vi "Remove Virtual Drive.vi"(8 "error in (no error)":errorcluster, 11 "BuildWorker Controller in":refnum<class "BuildWorker Controller.lvclass">) -> (0 "error out":errorcluster, 3 "BuildWorker Controller out":refnum<class "BuildWorker Controller.lvclass">)   [LabVIEW 2017, in "BuildWorker Controller.lvlib" / "BuildWorker Controller.lvclass"]
uses:
  BuildWorker Controller.lvclass
  BuildWorker Controller.lvclass/BuildWorker Controller.ctl
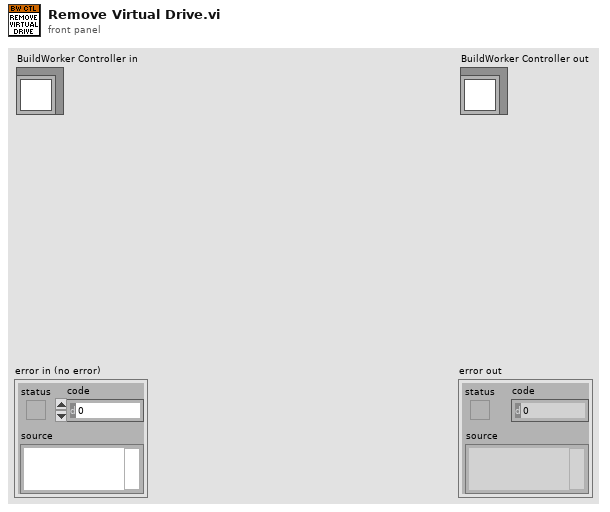
[diagram p1: front panel]
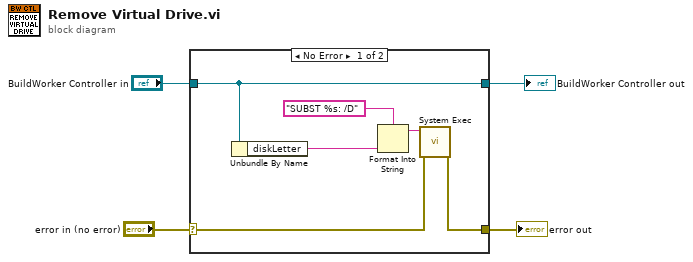
[diagram p0: block diagram]
diagram:
  n1 = case shown="No Error" "error in (no error)" {
    selector: "error in (no error)" -> [w6 w12]
    tunnel: [w5 w12] -> w1
    tunnel: [w10 w11] -> w3
    tunnel: "BuildWorker Controller in" -> [w10 w11]
    frame No Error {
      n2 = Unbundle By Name(w10) -> ("diskLetter"=w9:string)
      n3 = Format Into String(format string="SUBST %s: /D", w9) -> (resulting string=w7:string)  [unwired: 2 in, 1 out]
      n4 = call <vilib>:"System Exec.vi"("error in (no error)"=w6, "command line"=w7) -> ("error out"=w5:errorcluster)  [unwired: 6 in, 3 out]
    }
    frame Error {
    }
  }
  "error out" <- w1
  "BuildWorker Controller out" <- w3
